vi "TransferItems.vi"(8 "error in (no error)":errorcluster, 10 "Session":refnum<class "Session.lvclass">, 11 "TransferFolder-Put in":refnum<class "TransferFolder-Put.lvclass">) -> (0 "error out":errorcluster, 3 "TransferFolder-Put out":refnum<class "TransferFolder-Put.lvclass">)   [LabVIEW 2015, in "WinSCP.lvlib" / "TransferFolder-Put.lvclass"]
uses:
  TransferFolder-Put.lvclass
  Session/Session.lvclass
  C:/Users/Public/Documents/Projects/lv-winscp/Bin WinSCP/WinSCPnet.dll
  Bin WinSCP/WinSCPnet.dll
  FileTransferOptions/FileTransferOptions.lvclass
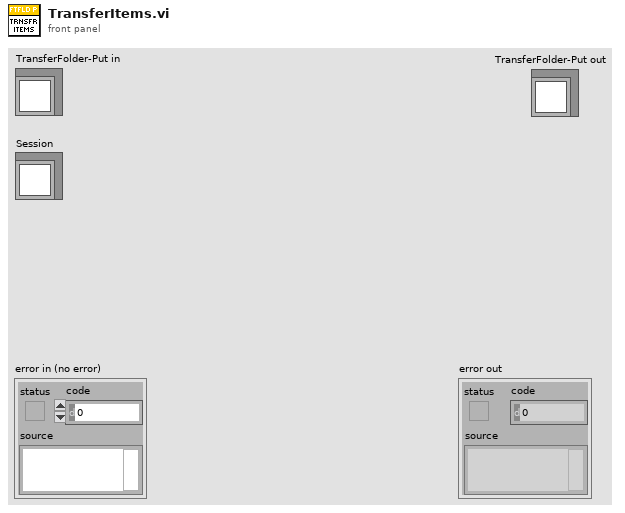
[diagram p1: front panel]
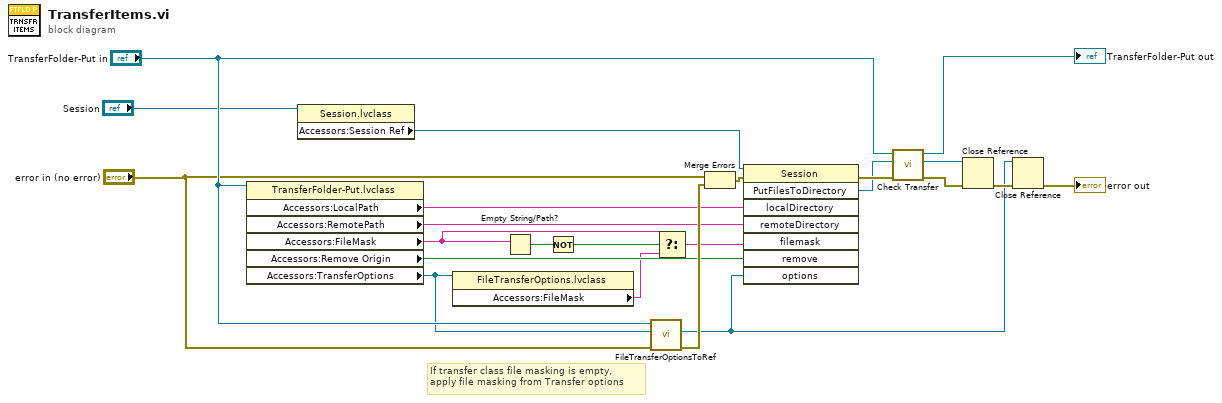
[diagram p0: block diagram]
diagram:
  # "If transfer class file masking is empty,\napply file masking from Transfer options"
  n1 = property class="TransferFolder-Put.lvclass"(reference="TransferFolder-Put in") -> ("Accessors:LocalPath"=w22:string, "Accessors:RemotePath"=w21:string, "Accessors:FileMask"=w4:string, "Accessors:Remove Origin"=w20:bool, "Accessors:TransferOptions"=w2:refnum<class "FileTransferOptions.lvclass">)  [unwired: 1 in, 2 out]
  n2 = property class="Session.lvclass"(reference="Session") -> ("Accessors:Session Ref"=w17:refnum<k24>)  [unwired: 1 in, 2 out]
  n3 = property class="FileTransferOptions.lvclass"(reference=w2) -> ("Accessors:FileMask"=w1:string)  [unwired: 1 in, 2 out]
  n4 = Empty String/Path?(string/path=w4) -> (empty?=w6:bool)
  n5 = Not(x=w6) -> (.not. x?=w5:bool)
  n6 = call-dynamic "FileTransferOptionsToRef.vi"("error in (no error)"="error in (no error)", "FileTransferOptions"=w2, "FileTransfer in"="TransferFolder-Put in") -> ("error out"=w23:errorcluster, "TransferOptions Ref"=w13:refnum<k24>)  [unwired: 7 in]
  n7 = Select(t=w4, s=w5, f=w1) -> (s? t:f=w3:string)
  n8 = Merge Errors("error in (no error)", w23) -> (w12:errorcluster)
  n9 = invoke class="Session" method="PutFilesToDirectory"(reference=w17, error in=w12, "localDirectory"=w22, "remoteDirectory"=w21, "filemask"=w3, "remove"=w20, "options"=w13) -> (error out=w19:errorcluster, "PutFilesToDirectory"=w18:refnum<k24>)  [unwired: 1 in, 6 out]
  n10 = call-dynamic "Check Transfer.vi"("error in"=w19, "TransferOperationResult in"=w18, "FileTransfer in"="TransferFolder-Put in") -> ("error out"=w15:errorcluster, "TransferOperationResult out"=w16:refnum<k24>, "FileTransfer out"=→"TransferFolder-Put out":refnum<class "TransferFolder-Put.lvclass">)  [unwired: 6 in]
  n11 = Close Reference(reference=w16, error in (no error)=w15) -> (error out=w14:errorcluster)
  n12 = Close Reference(reference=w13, error in (no error)=w14) -> (error out=→"error out":errorcluster)
